vi "User Message Received.vi"(0 "Module in":refnum<class "Module.lvclass">, 5 "Message":refnum<class "Message.lvclass">, 11 "Error in":errorcluster caption="Error in (no error)") -> (4 "Module out":refnum<class "Module.lvclass">, 15 "Error out":errorcluster)   [LabVIEW 2019, in "GP Module.lvlib" / "Module.lvclass"]
doc: "This VI runs whenever the Actor Core receives a message. Any messages not handled here are simply discarded.\n\n<B>You should not invoke the Call Parent Method node when adding this override.</B>\n\nSteen Schmidt\nGPower\n8/5 2017"
uses:
  Module.lvclass
  C:/Program Files (x86)/National Instruments/LabVIEW 2019/vi.lib/GPower/Actor/Library/Actor Class/Actor.lvclass
  <vilib>/GPower/Message/Library/Message Class/Message.lvclass
  <vilib>/GPower/Message/Library/Message Class/Message.lvclass/Message.ctl
  Module.lvclass/Module.ctl
  <vilib>/GPower/Actor/Library/Actor Class/Actor.lvclass/Actor.ctl
  <vilib>/GPower/Actor/Library/Actor Interface Class/Actor Interface.lvclass/Actor Interface.ctl
  <vilib>/GPower/Logger/Library/Logger Class/Logger.lvclass/Logger.ctl
  <vilib>/GPower/Logger/Library/Logger Class/Logger/Log.vi
  <vilib>/GPower/Actor/Library/Actor Interface Class/Accessors/Get Actor Name.vi
  <vilib>/GPower/Logger/Library/Logger Class/Accessors/Get Enabled State.vi
  <vilib>/GPower/Logger/Library/Logger Class/Accessors/Get Severity Level Threshold.vi
  <vilib>/GPower/Logger/Library/Logger Class/Logger/Promote.vi
  <vilib>/GPower/Logger/Library/Logger Class/Accessors/Get Error And Warning Promotion.vi
  <vilib>/GPower/Logger/Library/Logger Class/Logger.lvclass
  <vilib>/GPower/Actor/Library/Actor Class/Actor.lvclass
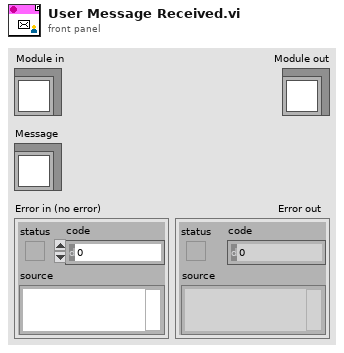
[diagram p1: front panel]
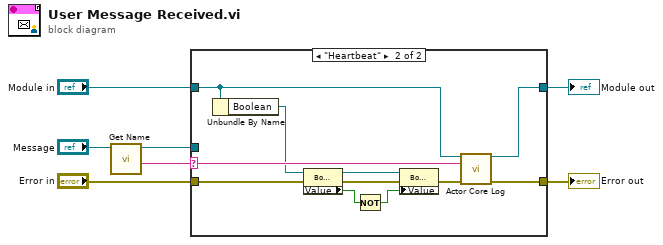
[diagram p0: block diagram]
diagram:
  n1 = call <vilib>:"Get Name.vi"("Message in"="Message") -> ("Name"=w5:string, "Message out"=w6:refnum<class "Message.lvclass">)  [unwired: 9 in]
  n2 = case shown="\"Heartbeat\"" w5 {
    selector: w5 -> [_ w18]
    tunnel: w6 -> [_ _]
    tunnel: "Module in" -> [w9 w17]
    tunnel: "Error in" -> [w8 w13]
    tunnel: [w8 w20] -> w2
    tunnel: [w9 w19] -> w1
    frame Default {
    }
    frame "Heartbeat" {
      n3 = Unbundle By Name(w17) -> ("Boolean"=w16:refnum<vi>)
      n4 = property class="Bool (strict)"(reference=w16, error in=w13) -> (reference out=w15:refnum<vi>, error out=w14:errorcluster, "Value"=w11:bool)
      n5 = Not(x=w11) -> (.not. x?=w10:bool)
      n6 = property class="Bool (strict)"(reference=w15, error in=w14, "Value"=w10) -> (error out=w12:errorcluster)  [unwired: 1 out]
      n7 = call <vilib>:"Actor Core Log.vi"("Actor in"=w17, "Log Message"=w18, "Error in"=w12) -> ("Actor out"=w19:refnum<class "Module.lvclass">, "Error out"=w20:errorcluster)  [unwired: 11 in]
    }
  }
  "Module out" <- w1
  "Error out" <- w2
